vi "Queue_Status (SubVI).vi"(8 "error in (no error)":errorcluster, 11 "Queue in":refnum<queue>) -> (0 "error out":errorcluster)   [LabVIEW 2017]
uses:
  Control_EU/DataCluster.ctl
  Control_EU/UNDT_ClusterPackRevers (Type).ctl
  Global_SNK3_HF.vi
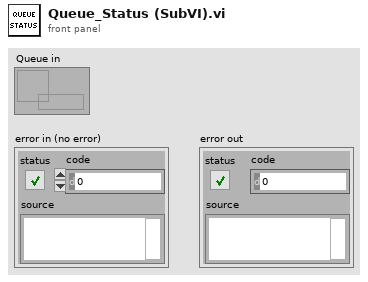
[diagram p1: front panel]
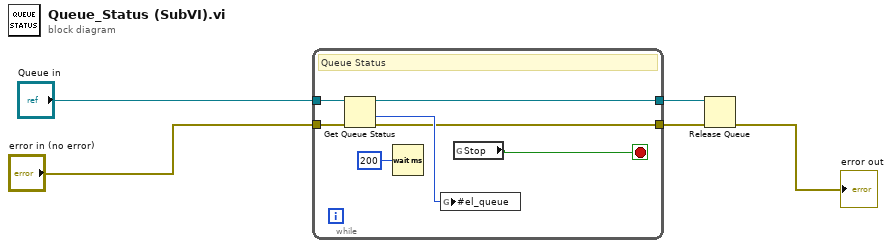
[diagram p0: block diagram]
diagram:
  n1 = while {
    tunnel: "Queue in" -> [w12]
    tunnel: [w6] -> w1
    tunnel: "error in (no error)" -> [w11]
    tunnel: [w10] -> w2
    stop <- w7 stop-if-true
    # "Queue Status"
    n2 = Get Queue Status(queue=w12, error in (no error)=w11) -> (queue out=w10:refnum<queue>, # pending insert=w8:i32, error out=w6:errorcluster)  [unwired: 6 out]
    n3 = Wait (ms)(milliseconds to wait=u32 200) -> ()  [unwired: 1 out]
    n4 = global write "Global_SNK3_HF.vi" "#el_queue"(w8) -> ()
    n5 = global read "Global_SNK3_HF.vi" "Stop"() -> (w7:bool)
  }
  n6 = Release Queue(queue=w2, error in (no error)=w1) -> (error out=→"error out":errorcluster)  [unwired: 3 out]
